vi "niFPGA Unit Delay_m.vi"   [LabVIEW 2017]
doc: "Delays the input value for one cycle. The data type you wire to <B>input</B> determines the <B>output</B> data type."
uses:
  <vilib>/rvi/Analysis/common/FxpNativeNode/niFpgaFxpNative.xnode
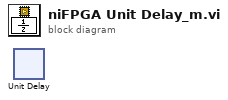
[diagram p0: block diagram]
diagram:
  n1 = xnode ("Unit Delay")() -> ()  [unwired: 3 in, 1 out]
